vi "单向脚本.vi"(0 "扫描电压(V)":dbl, 2 "电压改变量":dbl, 3 "极限电流(mA)":dbl min=0.0 max=50.0 step=0.1) -> (7 "Script":string)   [LabVIEW 2019]
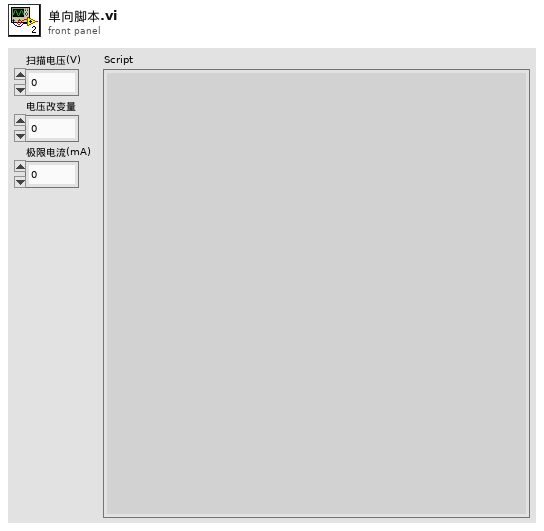
[diagram p1: front panel]
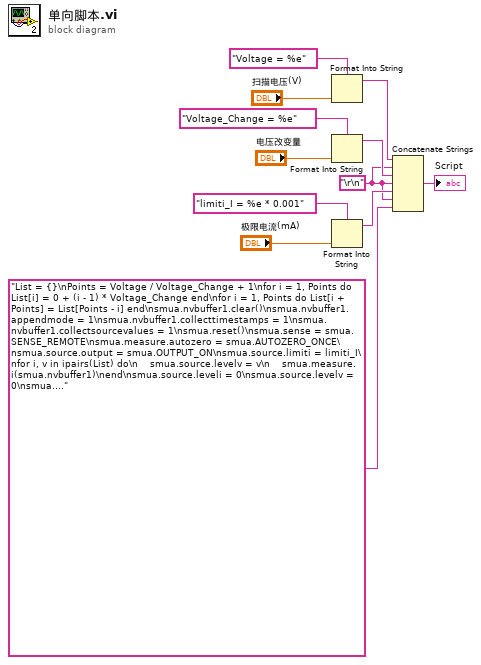
[diagram p0: block diagram]
diagram:
  w3 = "\r\n"
  n1 = Format Into String(format string="Voltage = %e" ("格式字符串"), "扫描电压(V)") -> (resulting string=w7:string)  [unwired: 2 in, 1 out]
  n2 = Format Into String(format string="Voltage_Change = %e" ("格式字符串"), "电压改变量") -> (resulting string=w5:string)  [unwired: 2 in, 1 out]
  n3 = Format Into String(format string="limiti_I = %e * 0.001" ("格式字符串"), "极限电流(mA)") -> (resulting string=w4:string)  [unwired: 2 in, 1 out]
  n4 = Concatenate Strings(w7, w3, w5, w3, w4, w3, "List = {}\nPoints = Voltage / Voltage_Change + 1\nfor i = 1, Points do List[i] = 0 + (i - 1) * Voltage_Change end\nfor i = 1, Points do List[i + Points] = List[Points - i] end\nsmua.nvbuffer1.clear()\nsmua.nvbuffer1.appendmode = 1\nsmua.nvbuffer1.collecttimestamps = 1\nsmua.nvbuffer1.collectsourcevalues = 1\nsmua.reset()\nsmua.sense = smua.SENSE_REMOTE\nsmua.measure.autozero = smua.AUTOZERO_ONCE\nsmua.source.output = smua.OUTPUT_ON\nsmua.source.limiti = limiti_I\nfor i, v in ipairs(List) do\n    smua.source.levelv = v\n    smua.measure.i(smua.nvbuffer1)\nend\nsmua.source.leveli = 0\nsmua.source.levelv = 0\nsmua.source.output = smua.OUTPUT_OFF\nprint(\"{done}\")\nreset()") -> (→"Script":string)
